vi "power_of_2.vi"(11 "x":dbl) -> (3 "2^x":dbl)   [LabVIEW 2019]
panel:
  out "error out":errorcluster
  in  "error in":errorcluster
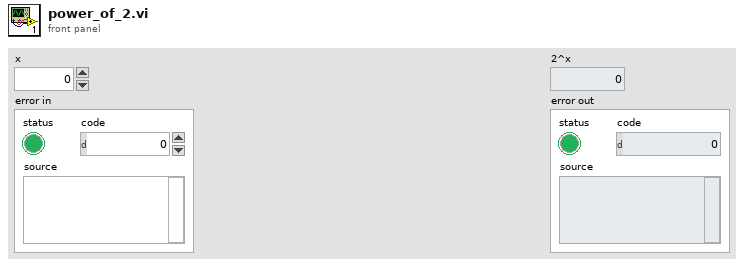
[diagram p1: front panel]
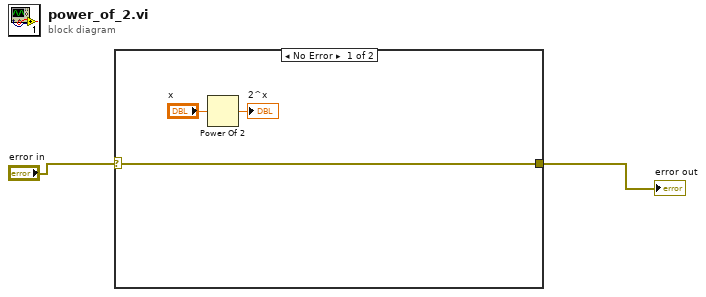
[diagram p0: block diagram]
diagram:
  n1 = case shown="No Error" "error in" {
    selector: "error in" -> [w3 w6]
    tunnel: [w3 w6] -> w1
    frame No Error {
      n2 = Power Of 2(x="x") -> (2^x=→"2^x":dbl)
    }
    frame Error {
    }
  }
  "error out" <- w1
